vi "GetParam.vi"(8 "error in (no error)":errorcluster caption="entrée d'erreur (pas d'erreur)", 11 "Matthews_Corrcoef.lvclass":refnum<class "Matthews_Corrcoef.lvclass">) -> (0 "error out":errorcluster caption="sortie d'erreur", 2 "matthews_corrcoef":cluster{"sample_weight":dbl[]}, 3 "Matthews_Corrcoef.lvclass":refnum<class "Matthews_Corrcoef.lvclass">)   [LabVIEW 2020, in "Matthews_Corrcoef.lvclass"]
doc: "Get Parameters"
uses:
  Matthews_Corrcoef.lvclass
  Matthews_Corrcoef.lvclass/Matthews_Corrcoef.ctl
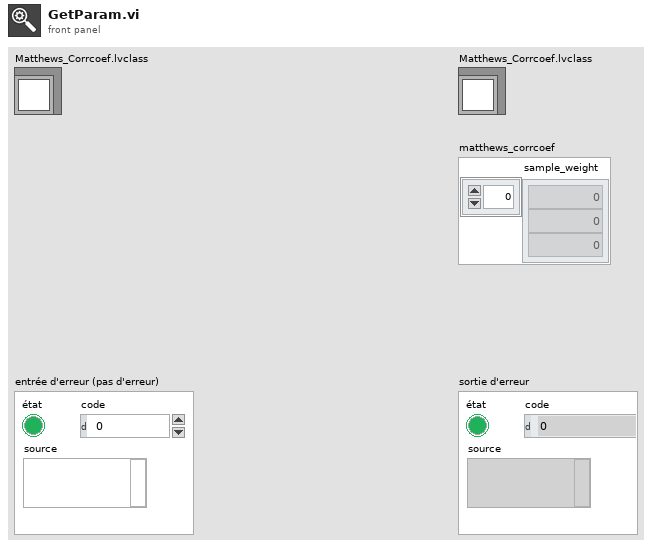
[diagram p1: front panel]
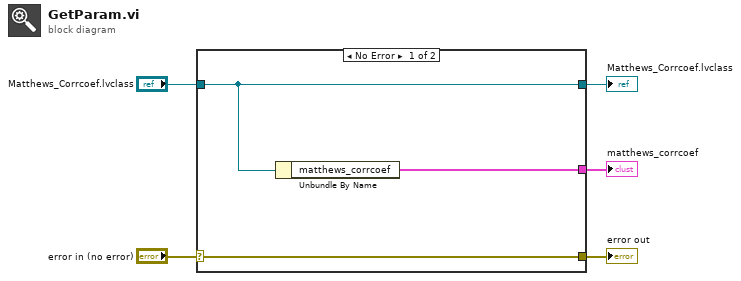
[diagram p0: block diagram]
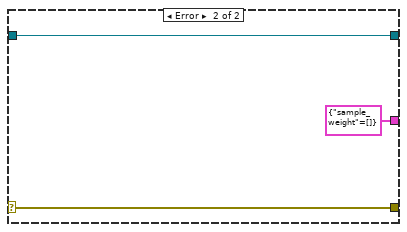
[diagram p2: hidden frame]
diagram:
  n1 = case shown="No Error" "error in (no error)" {
    selector: "error in (no error)" -> [w8 w10]
    tunnel: [w8 w10] -> w4
    tunnel: [w7 w11] -> w2
    tunnel: "Matthews_Corrcoef.lvclass" -> [w7 w11]
    tunnel: [w6 cluster{"sample_weight":dbl[]} {"sample_weight"=[]} ("matthews_corrcoef")] -> w1
    frame No Error {
      n2 = Unbundle By Name(w7) -> ("matthews_corrcoef"=w6:cluster{"sample_weight":dbl[]})
    }
    frame Error {
    }
  }
  "error out" <- w4
  "Matthews_Corrcoef.lvclass" <- w2
  "matthews_corrcoef" <- w1
